vi "Toggle Defer.vi"(6 "Defer":bool, 8 "error in":errorcluster, 11 "Report Viewer in":refnum<class "Report Viewer.lvclass">) -> (0 "error out":errorcluster, 3 "Report Viewer out":refnum<class "Report Viewer.lvclass">)   [LabVIEW 2023, in "Report Viewer.lvlib" / "Report Viewer.lvclass"]
uses:
  Library/Report Viewer.lvclass
  C:/Users/Public/Documents/Development/builds/Engine/Engine.lvlibp/Project/Engine.lvclass
  builds/Engine/Engine.lvlibp/Accessors/Read VI_Ref.vi
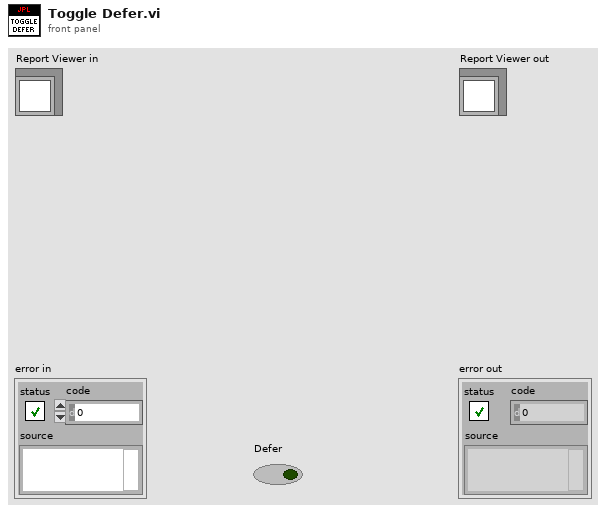
[diagram p1: front panel]
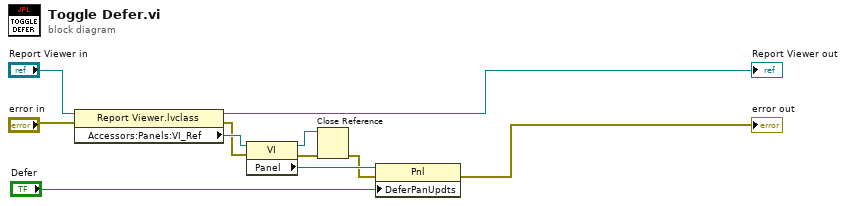
[diagram p0: block diagram]
diagram:
  n1 = property class="Report Viewer.lvclass"(reference="Report Viewer in", error in="error in") -> (reference out=→"Report Viewer out":refnum<class "Report Viewer.lvclass">, error out=w1:errorcluster, "Accessors:Panels:VI_Ref"=w2:refnum<vi>)
  n2 = property class="VI"(reference=w2, error in=w1) -> (reference out=w11:refnum<vi>, error out=w10:errorcluster, "Panel"=w9:refnum<vi>)
  n3 = Close Reference(reference=w11, error in (no error)=w10) -> (error out=w7:errorcluster)
  n4 = property class="Pnl"(reference=w9, error in=w7, "DeferPanUpdts"="Defer") -> (error out=→"error out":errorcluster)  [unwired: 1 out]
